vi "Clean Closing Sign from Pointer String.vi"(10 "String In":string) -> (2 "String Out":string)   [LabVIEW 2012]
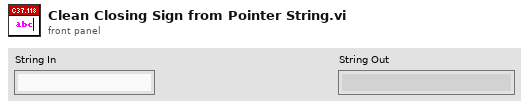
[diagram p1: front panel]
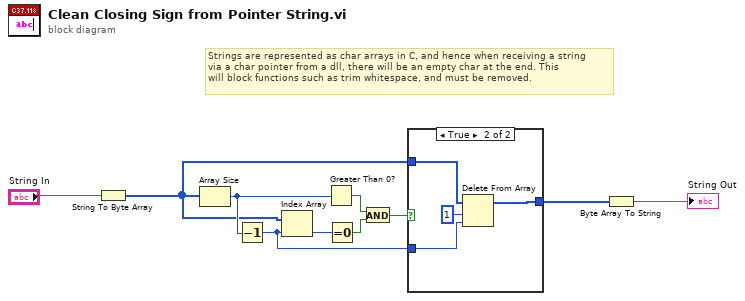
[diagram p0: block diagram]
diagram:
  # "Strings are represented as char arrays in C, and hence when receiving a string\nvia a char pointer from a dll, there will be an empty char at the end. This\nwill block functions such as trim whitespace, and must be removed."
  n1 = String To Byte Array(string="String In") -> (unsigned byte array=w7:u8[])
  n2 = Array Size(array=w7) -> (size(s)=w8:i32)
  n3 = Decrement(x=w8) -> (x-1=w3:i32)
  n4 = Index Array(array=w7, index=w3) -> (element=w9:u8)
  n5 = Greater Than 0?(x=w8) -> (x > 0?=w5:bool)
  n6 = Equal To 0?(x=w9) -> (x = 0?=w6:bool)
  n7 = And(x=w5, y=w6) -> (x .and. y?=w4:bool)
  n8 = case shown="True" w4 {
    tunnel: w7 -> [w11 w15]
    tunnel: w3 -> [_ w14]
    tunnel: [w11 w12] -> w2
    frame False {
    }
    frame True {
      n9 = Delete From Array(array=w15, length=1, index=w14) -> (array with subset deleted=w12:u8[])  [unwired: 1 out]
    }
  }
  n10 = Byte Array To String(unsigned byte array=w2) -> (string=→"String Out":string)
